vi "Readout_Spectrum_old.vi"(0 "tdms file in":refnum<k34>, 5 "Ch1_in":dbl[](array[numeric]), 7 "Ch2_in":dbl[](array[numeric]), 9 "Ch3_in":dbl[](array[numeric]), 11 "Ch4_in":dbl[](array[numeric]), 12 "group name":string, 13 "channel names":string[](array[string])) -> (4 "tdms file out":refnum<k34>, 6 "Ch1_out":dbl[](array[numeric]), 8 "Ch2_out":dbl[](array[numeric]), 10 "Ch3_out":dbl[](array[numeric]), 14 "Spectrum":T1(array[cluster]), 15 "Ch4_out":dbl[](array[numeric]))   [LabVIEW 2019]
uses:
  SiPM_Tests_Global_Var.vi
  Agilent_lib/Public/Data/Read Measurement (Current Value).vi
  Agilent_lib/Agilent 2000 3000 X-Series.lvlib
  <vilib>/Analysis/NI_AALPro.lvlib
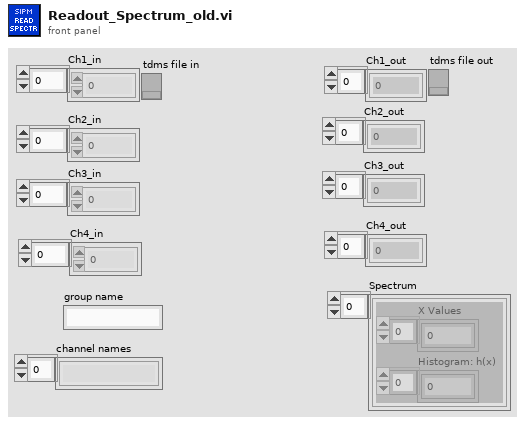
[diagram p1: front panel]
types:
  T1 = cluster{"X Values":dbl[], "Histogram: h(x)":i32[]}[]
  T2 = cluster{"X Values":dbl[], "Histogram: h(x)":i32[]}
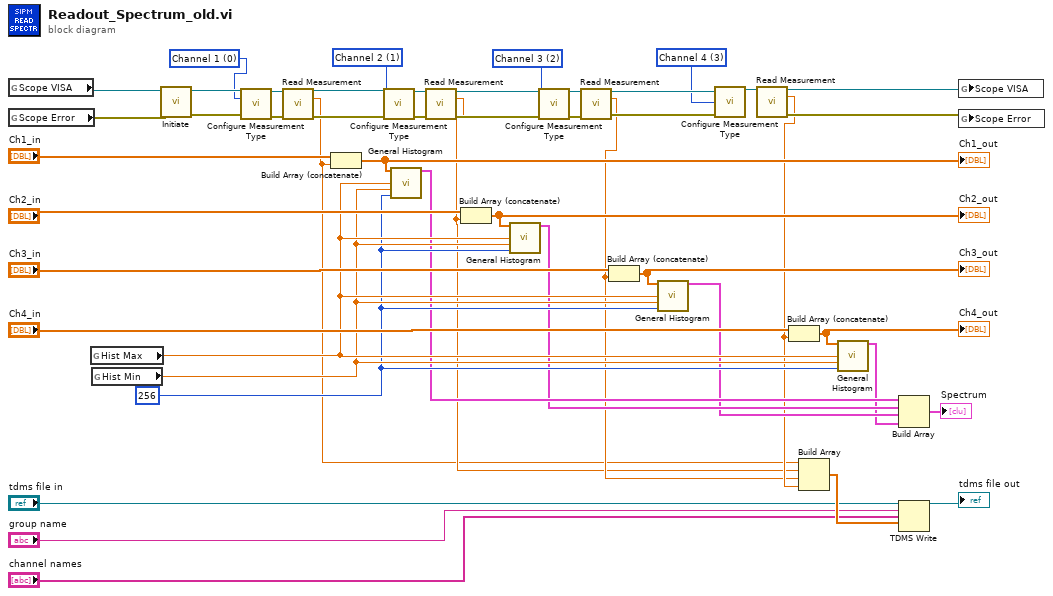
[diagram p0: block diagram]
diagram:
  w28 = 0 items=["Channel 1"=0, "Channel 2"=1, "Channel 3"=2, "Channel 4"=3, "Math"=4, "Waveform Memory 1"=5, "Waveform Memory 2"=6, "D0"=13, "D1"=14, "D2"=15, "D3"=16, "D4"=17, "D5"=18, "D6"=19, "D7"=20, "D8"=21, "D9"=22, "D10"=23, "D11"=24, "D12"=25, "D13"=26, "D14"=27, "D15"=28, "External"=29, "Function"=32] ("Measurement Source 1 (0: Channel 1)")
  w29 = 3 items=["Channel 1"=0, "Channel 2"=1, "Channel 3"=2, "Channel 4"=3, "Math"=4, "Waveform Memory 1"=5, "Waveform Memory 2"=6, "D0"=13, "D1"=14, "D2"=15, "D3"=16, "D4"=17, "D5"=18, "D6"=19, "D7"=20, "D8"=21, "D9"=22, "D10"=23, "D11"=24, "D12"=25, "D13"=26, "D14"=27, "D15"=28, "External"=29, "Function"=32] ("Measurement Source 1 (0: Channel 1)")
  w17 = 256 ("# bins")
  w44 = 2 items=["Channel 1"=0, "Channel 2"=1, "Channel 3"=2, "Channel 4"=3, "Math"=4, "Waveform Memory 1"=5, "Waveform Memory 2"=6, "D0"=13, "D1"=14, "D2"=15, "D3"=16, "D4"=17, "D5"=18, "D6"=19, "D7"=20, "D8"=21, "D9"=22, "D10"=23, "D11"=24, "D12"=25, "D13"=26, "D14"=27, "D15"=28, "External"=29, "Function"=32] ("Measurement Source 1 (0: Channel 1)")
  w39 = 1 items=["Channel 1"=0, "Channel 2"=1, "Channel 3"=2, "Channel 4"=3, "Math"=4, "Waveform Memory 1"=5, "Waveform Memory 2"=6, "D0"=13, "D1"=14, "D2"=15, "D3"=16, "D4"=17, "D5"=18, "D6"=19, "D7"=20, "D8"=21, "D9"=22, "D10"=23, "D11"=24, "D12"=25, "D13"=26, "D14"=27, "D15"=28, "External"=29, "Function"=32] ("Measurement Source 1 (0: Channel 1)")
  n1 = global read "SiPM_Tests_Global_Var.vi" "Scope VISA"() -> (w45:refnum<visa-resource-name>)
  n2 = global read "SiPM_Tests_Global_Var.vi" "Scope Error"() -> (w46:errorcluster)
  n3 = global read "SiPM_Tests_Global_Var.vi" "Hist Max"() -> (w19:dbl)
  n4 = global read "SiPM_Tests_Global_Var.vi" "Hist Min"() -> (w18:dbl)
  n5 = call "Initiate.vi"("error in (no error)"=w46, "VISA resource name"=w45) -> ("error out"=w47:errorcluster, "VISA resource name out"=w48:refnum<visa-resource-name>)  [unwired: 8 in]
  n6 = call "Configure Measurement Type.vi"("VISA resource name"=w48, "Measurement Type (0: Peak-Peak)"=w28, "error in (no error)"=w47) -> ("VISA resource name out"=w33:refnum<visa-resource-name>, "error out"=w34:errorcluster)  [unwired: 11 in]
  n7 = call-poly "Read Measurement.vi"("VISA resource name"=w33, "error in (no error)"=w34) -> ("VISA resource name out"=w36:refnum<visa-resource-name>, "Result Value"=w7:dbl, "error out"=w37:errorcluster)  [unwired: 11 in]
  n8 = Build Array (concatenate)("Ch1_in", w7) -> (w26:dbl[])
  "Ch1_out" <- w26
  n9 = call "Configure Measurement Type.vi"("VISA resource name"=w36, "Measurement Source 1 (0: Channel 1)"=w39, "error in (no error)"=w37) -> ("VISA resource name out"=w38:refnum<visa-resource-name>, "error out"=w35:errorcluster)  [unwired: 11 in]
  n10 = call <vilib>:"General Histogram.vi"("X"=w26, "max"=w19, "min"=w18, "# bins"=w17) -> ("Histogram Graph"=w16:T2)  [unwired: 7 in, 4 out]
  n11 = call-poly "Read Measurement.vi"("VISA resource name"=w38, "error in (no error)"=w35) -> ("VISA resource name out"=w40:refnum<visa-resource-name>, "Result Value"=w8:dbl, "error out"=w41:errorcluster)  [unwired: 11 in]
  n12 = Build Array (concatenate)("Ch2_in", w8) -> (w25:dbl[])
  "Ch2_out" <- w25
  n13 = call <vilib>:"General Histogram.vi"("X"=w25, "max"=w19, "min"=w18, "# bins"=w17) -> ("Histogram Graph"=w15:T2)  [unwired: 7 in, 4 out]
  n14 = call "Configure Measurement Type.vi"("VISA resource name"=w40, "Measurement Source 1 (0: Channel 1)"=w44, "error in (no error)"=w41) -> ("VISA resource name out"=w42:refnum<visa-resource-name>, "error out"=w43:errorcluster)  [unwired: 11 in]
  n15 = call-poly "Read Measurement.vi"("VISA resource name"=w42, "error in (no error)"=w43) -> ("VISA resource name out"=w31:refnum<visa-resource-name>, "Result Value"=w9:dbl, "error out"=w30:errorcluster)  [unwired: 11 in]
  n16 = Build Array (concatenate)("Ch3_in", w9) -> (w22:dbl[])
  "Ch3_out" <- w22
  n17 = call <vilib>:"General Histogram.vi"("X"=w22, "max"=w19, "min"=w18, "# bins"=w17) -> ("Histogram Graph"=w14:T2)  [unwired: 7 in, 4 out]
  n18 = call "Configure Measurement Type.vi"("VISA resource name"=w31, "Measurement Source 1 (0: Channel 1)"=w29, "error in (no error)"=w30) -> ("VISA resource name out"=w32:refnum<visa-resource-name>)  [unwired: 11 in, 1 out]
  n19 = call-poly "Read Measurement.vi"("VISA resource name"=w32) -> ("VISA resource name out"=w12:refnum<visa-resource-name>, "Result Value"=w10:dbl, "error out"=w11:errorcluster)  [unwired: 12 in]
  n20 = Build Array (concatenate)("Ch4_in", w10) -> (w20:dbl[])
  "Ch4_out" <- w20
  n21 = Build Array(w7, w8, w9, w10) -> (w6:dbl[])
  n22 = call <vilib>:"General Histogram.vi"("X"=w20, "max"=w19, "min"=w18, "# bins"=w17) -> ("Histogram Graph"=w13:T2)  [unwired: 7 in, 4 out]
  n23 = Build Array(w16, w15, w14, w13) -> (→"Spectrum":T1)
  n24 = TDMS Write(0:"tdms file in", 5:"group name", 7:"channel names", 9:w6) -> (4:→"tdms file out":refnum<k34>)  [unwired: 2 in, 3 out]
  n25 = global write "SiPM_Tests_Global_Var.vi" "Scope VISA"(w12) -> ()
  n26 = global write "SiPM_Tests_Global_Var.vi" "Scope Error"(w11) -> ()
